vi "Configure.vi"(8 "error in (no error)":errorcluster, 11 "Thorcam in":refnum<class "Thorcam.lvclass">) -> (0 "error out":errorcluster, 2 "cancelled?":bool, 3 "Thorcam out":refnum<class "Thorcam.lvclass">)   [LabVIEW 2012, in "Thorcam.lvclass"]
doc: "The configure method configures the details for the RabbitMQ connection, the observers and the mapping script.\n\nIn the derived class, make a call to the parent for setting these parameters."
uses:
  Thorcam.lvclass
  cross correlation method.ctl
  <vilib>/Utility/miscctls.llb/LVPointTypeDef.ctl
  Thorcam.lvclass/Thorcam.ctl
  <vilib>/Distrio/Murmex/Murmex/Murmex.lvclass
panel:
  in  "Tab Control":T1(tab)
  in  "2nd camera ID":u32
  in  "Settings":string
  in  "1st camera ID":u32
  in  "Background":path
  in  "Alignment quality threshold":dbl
  in  "Shift to defocus conversion factor":dbl
  in  "Stage component":string
  in  "LUT":path
  in  "File path to save images":path
  in  "Cross Correlation method":T2
  in  "button:cancel":bool
  in  "button:call parent":bool
  in  "button:ok":bool
  # "RabbitMQ parameters"
  # "Window position"
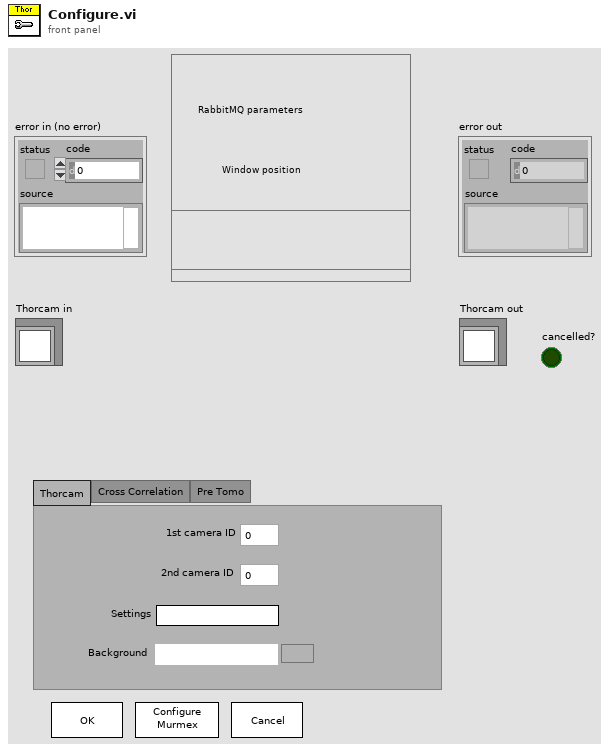
[diagram p1: front panel]
types:
  T1 = enum32{"Thorcam", "Cross Correlation", "Pre Tomo"}
  T2 = typedef "Thorcam.lvclass/cross correlation method.ctl" = enum16{"default", "normalised cross correlation", "normalised mutual information", "binary cross correlation"}
  T3 = typedef "LVPointTypeDef.ctl" = cluster{"Horizontal":i16, "Vertical":i16}
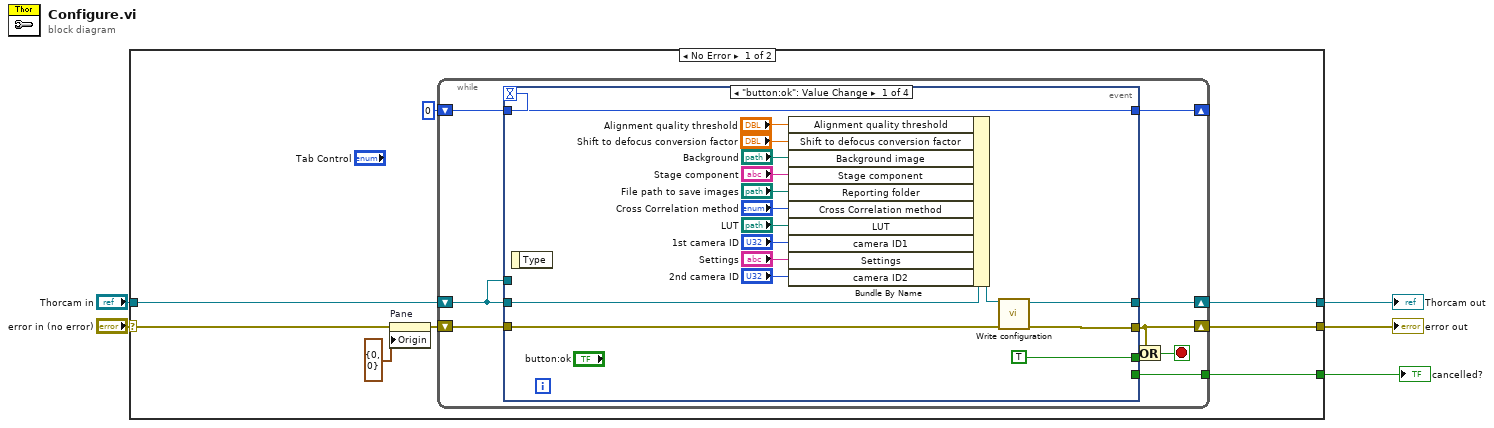
[diagram p0: block diagram]
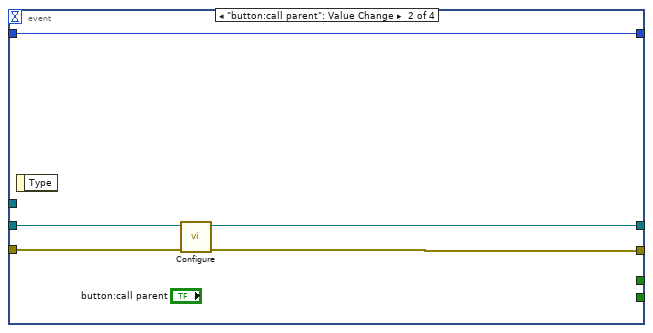
[diagram p2: hidden frame]
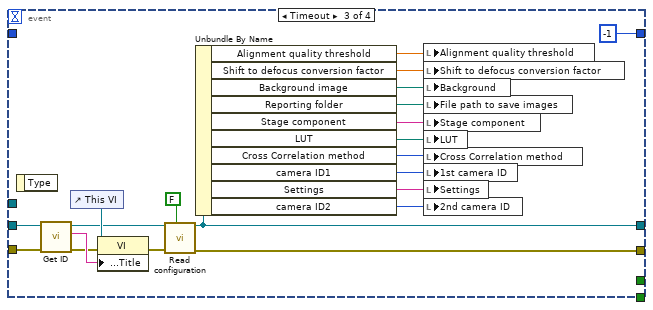
[diagram p3: hidden frame]
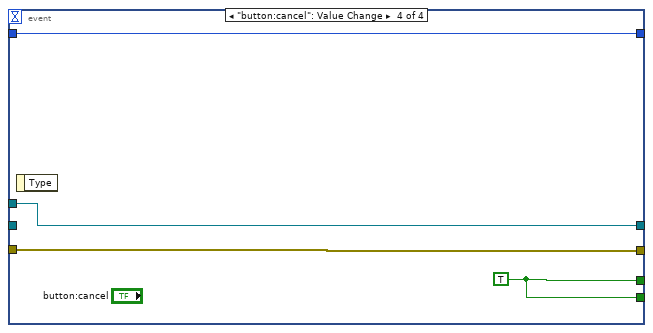
[diagram p4: hidden frame]
diagram:
  n1 = case shown="No Error" "error in (no error)" {
    selector: "error in (no error)" -> [w12 w70]
    tunnel: "Thorcam in" -> [w10 w71]
    tunnel: [w9 w70] -> w3
    tunnel: [w8 w71] -> w2
    tunnel: [w7 _] -> w1
    frame No Error {
      n2 = property on="Pane" class="Pane"(error in=w12, "Origin"=T3 {"Horizontal"=0, "Vertical"=0}) -> (error out=w11:errorcluster)  [unwired: 1 in, 1 out]
      n3 = while {
        shift-right: [w16] -> _
        shift-left: 0 -> [w21]
        shift-right: [w19] -> w9
        shift-left: w11 -> [w22]
        shift-right: [w20] -> w8
        shift-left: w10 -> [w14]
        tunnel: [w15] -> w7
        stop <- w17 stop-if-true
        n4 = event shown="[0] \"button:ok\": Value Change" {
          selector: _ -> [_ _ _ _]
          dyn-events: _ -> [_ _ _ _]
          timeout: w21 -> [_ _ _ _]
          tunnel: w21 -> [w33 w44 _ w69]
          tunnel: w22 -> [w35 w43 w60 w66]
          tunnel: w14 -> [w37 w41 w61 _]
          tunnel: [w39 w42 w47 w66] -> w19
          tunnel: [w38 w40 w48 w67] -> w20
          tunnel: [TRUE ("cancelled?") _ _ w68] -> w18
          tunnel: [w33 w44 -1 w69] -> w16
          tunnel: [_ _ _ w68] -> w15
          tunnel: w14 -> [_ _ _ w67]
          event "button:ok": Value Change {
            n5 = event-data() -> ()  [unwired: 1 in, 1 out]
            n6 = Bundle By Name(cluster=w37, "Alignment quality threshold"="Alignment quality threshold", "Shift to defocus conversion factor"="Shift to defocus conversion factor", "Background image"="Background", "Stage component"="Stage component", "Reporting folder"="File path to save images", "Cross Correlation method"="Cross Correlation method", "LUT"="LUT", "camera ID1"="1st camera ID", "Settings"="Settings", "camera ID2"="2nd camera ID") -> (w36:refnum<class "Thorcam.lvclass">)
            n7 = call-dynamic "Write configuration.vi"("error in (no error)"=w35, "Thorcam in"=w36) -> ("error out"=w39:errorcluster, "Thorcam out"=w38:refnum<class "Thorcam.lvclass">)  [unwired: 8 in]
          }
          event "button:call parent": Value Change {
            n8 = event-data() -> ()  [unwired: 1 in, 1 out]
            n9 = call-parent "Configure.vi"("error in (no error)"=w43, "Murmex in"=w41) -> ("error out"=w42:errorcluster, "Murmex out"=w40:refnum<class "Thorcam.lvclass">)  [unwired: 7 in, 1 out]
          }
          event Timeout {
            n10 = event-data() -> ()  [unwired: 1 in, 1 out]
            n11 = call <vilib>:"Get ID.vi"("error in (no error)"=w60, "Murmex in"=w61) -> ("error out"=w62:errorcluster, "component id"=w64:string, "Murmex out"=w59:refnum<class "Thorcam.lvclass">)  [unwired: 7 in]
            n12 = control-ref of="This VI"() -> (w63:refnum<vi>)
            n13 = property class="VI"(reference=w63, error in=w62, "Front Panel.Title"=w64) -> (error out=w58:errorcluster)  [unwired: 1 out]
            n14 = call-dynamic "Read configuration.vi"("force loading?"=FALSE, "error in (no error)"=w58, "Thorcam in"=w59) -> ("error out"=w47:errorcluster, "Thorcam out"=w48:refnum<class "Thorcam.lvclass">)  [unwired: 7 in]
            n15 = Unbundle By Name(w48) -> ("Alignment quality threshold"=w45:dbl, "Shift to defocus conversion factor"=w46:dbl, "Background image"=w50:path, "Reporting folder"=w51:path, "Stage component"=w52:string, "LUT"=w53:path, "Cross Correlation method"=w54:T2, "camera ID1"=w56:u32, "Settings"=w55:string, "camera ID2"=w49:u32)
            n16 = local write "Alignment quality threshold"(w45) -> ()
            n17 = local write "Shift to defocus conversion factor"(w46) -> ()
            n18 = local write "Background"(w50) -> ()
            n19 = local write "File path to save images"(w51) -> ()
            n20 = local write "Stage component"(w52) -> ()
            n21 = local write "LUT"(w53) -> ()
            n22 = local write "Cross Correlation method"(w54) -> ()
            n23 = local write "1st camera ID"(w56) -> ()
            n24 = local write "Settings"(w55) -> ()
            n25 = local write "2nd camera ID"(w49) -> ()
          }
          event "button:cancel": Value Change {
            w68 = TRUE ("cancelled?")
            n26 = event-data() -> ()  [unwired: 1 in, 1 out]
          }
        }
        n27 = Or(x=w19, y=w18) -> (x .or. y?=w17:bool)
      }
    }
    frame Error {
    }
  }
  "error out" <- w3
  "Thorcam out" <- w2
  "cancelled?" <- w1
